vi "ECU ADC Test.vi"(5 "Socket":u32, 6 "Wait (ms)":u32, 7 "LookupTable":refnum<data-value>, 9 "Connection Ref":refnum<k5>, 10 "Expected Value":dbl, 11 "PinName":string) -> (0 "error out":errorcluster, 1 "Connection Ref out":refnum<k5>, 2 "Report Text":string, 3 "Measurement":dbl)   [LabVIEW 2024, in "Shared Steps.lvlib"]
uses:
  Shared Steps.lvlib
  Types/Pin Mapping.ctl
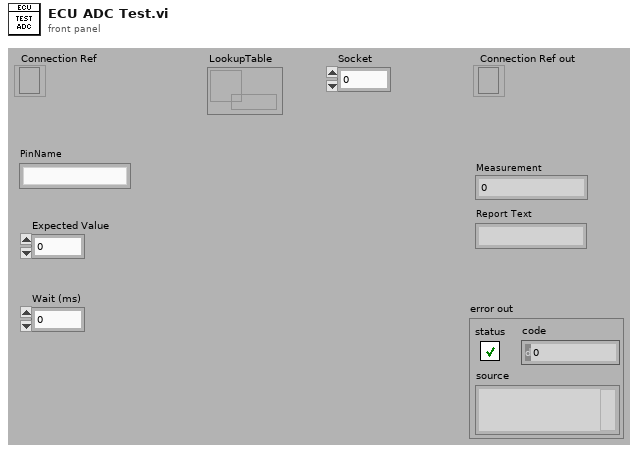
[diagram p1: front panel]
types:
  T1 = typedef "Shared Steps.lvlib/Pin Mapping.ctl" = cluster{"DUT":string, "ECU Pin Name":string, "Device Pin Name":string, "ECU Signal Type":string, "ECU Signal Direction":string, "MessageID":string}
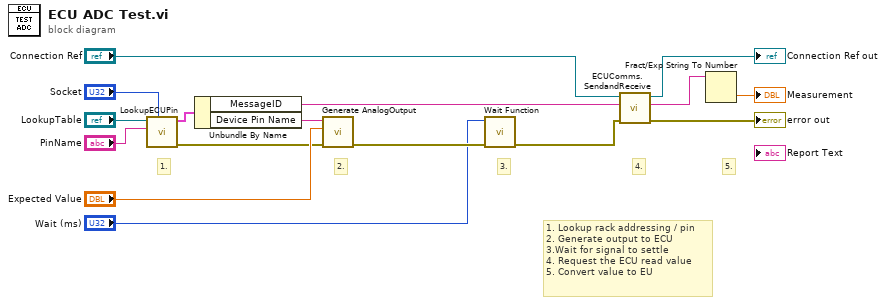
[diagram p0: block diagram]
diagram:
  # "1. Lookup rack addressing / pin\n2. Generate output to ECU\n3.Wait for signal to settle\n4. Request the ECU read value\n5. Convert value to EU"
  # "5."
  # "4."
  # "3."
  # "2."
  # "1."
  n1 = call "LookupECUPin.vi"("Socket"="Socket", "ECU Pin"="PinName", "LookupTable"="LookupTable") -> ("error out"=w3:errorcluster, "Info"=w14:T1)  [unwired: 6 in, 1 out]
  n2 = Unbundle By Name(w14) -> ("MessageID"=w10:string, "Device Pin Name"=w12:string)
  n3 = call "Generate AnalogOutput.vi"("error in (no error)"=w3, "Output Value"="Expected Value", "Rack Pin"=w12) -> ("error out"=w6:errorcluster)  [unwired: 8 in]
  n4 = call "Wait Function.vi"("error in (no error)"=w6, "Wait (ms)"="Wait (ms)") -> ("error out"=w5:errorcluster)  [unwired: 9 in]
  n5 = call "ECUComms.SendandReceive.vi"("error in (no error)"=w5, "Request ID"=w10, "Connection Ref"="Connection Ref") -> ("error out"=→"error out":errorcluster, "Response"=w2:string, "Connection Ref out"=→"Connection Ref out":refnum<k5>)  [unwired: 6 in]
  n6 = Fract/Exp String To Number(string=w2) -> (number=→"Measurement":dbl)  [unwired: 3 in, 1 out]
